vi "Special_Processing.vi"(6 "cluster in":T1, 8 "error in (no error)":errorcluster, 9 "Terminal Map In":map{string, T3}(c390), 10 "Wires":T2[](array[typedef]), 11 "GrowableObjectFunction in":refnum<class "PropertyNode.lvclass">) -> (0 "error out":errorcluster, 1 "Terminal Map Out":map{string, T3}(c390), 2 "Wires out":T2[](array[typedef]), 3 "GrowableObjectFunction out":refnum<class "PropertyNode.lvclass">)   [LabVIEW 2025, in "PropertyNode.lvclass"]
uses:
  PropertyNode.lvclass
  wire.ctl
  Terminal.ctl
  bd.ctl
  Node/Node.lvclass
  Node/Node.lvclass/Node.ctl
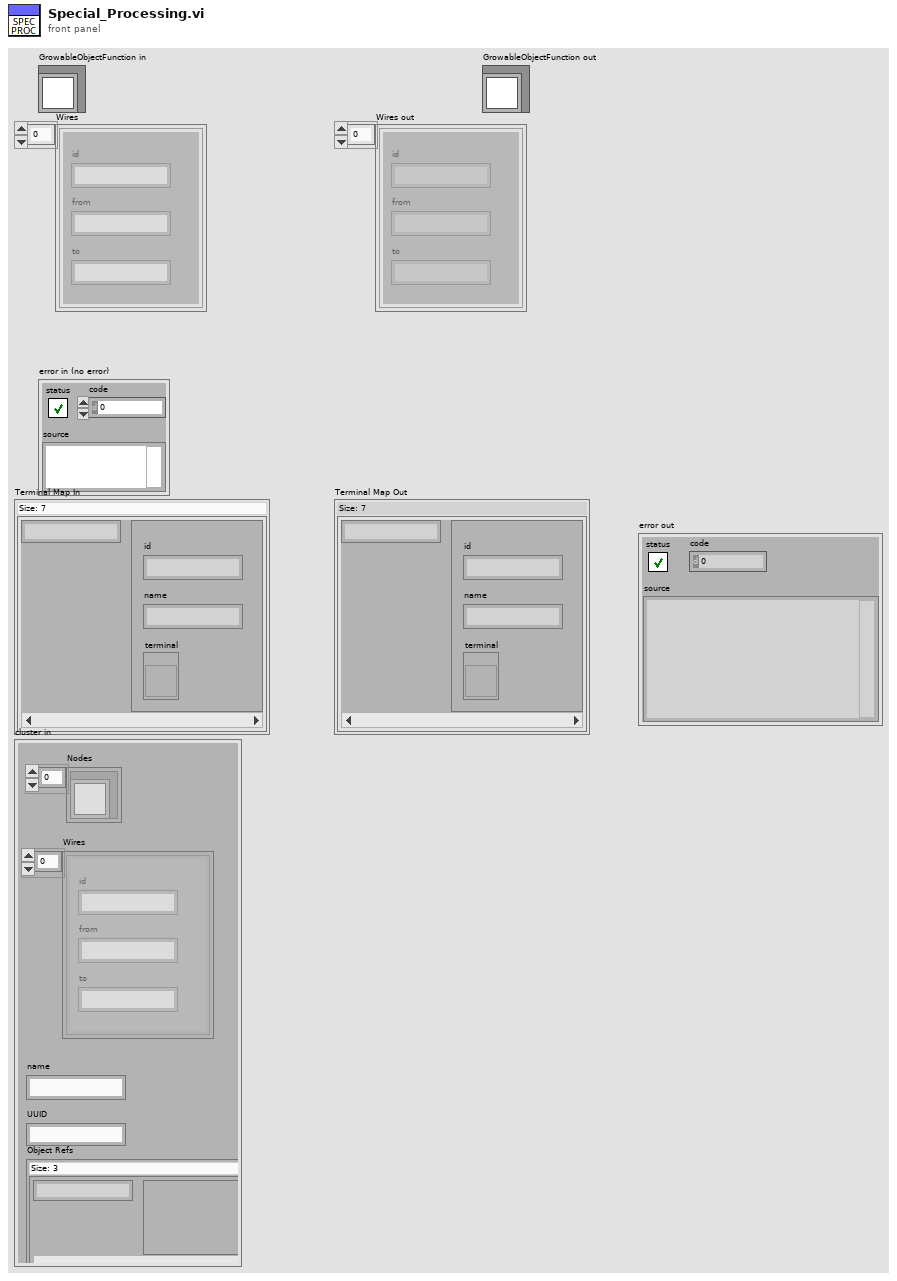
[diagram p1: front panel]
types:
  T1 = typedef "bd.ctl" = cluster{"Nodes":refnum<class "Node.lvclass">[], "Wires":T2[], "name":string, "UUID":string, "Object Refs":map{string, variant}}
  T2 = typedef "wire.ctl" = cluster{"id":string, "from":string, "to":string}
  T3 = typedef "Terminal.ctl" = cluster{"id":string, "name":string, "terminal":refnum<vi>}
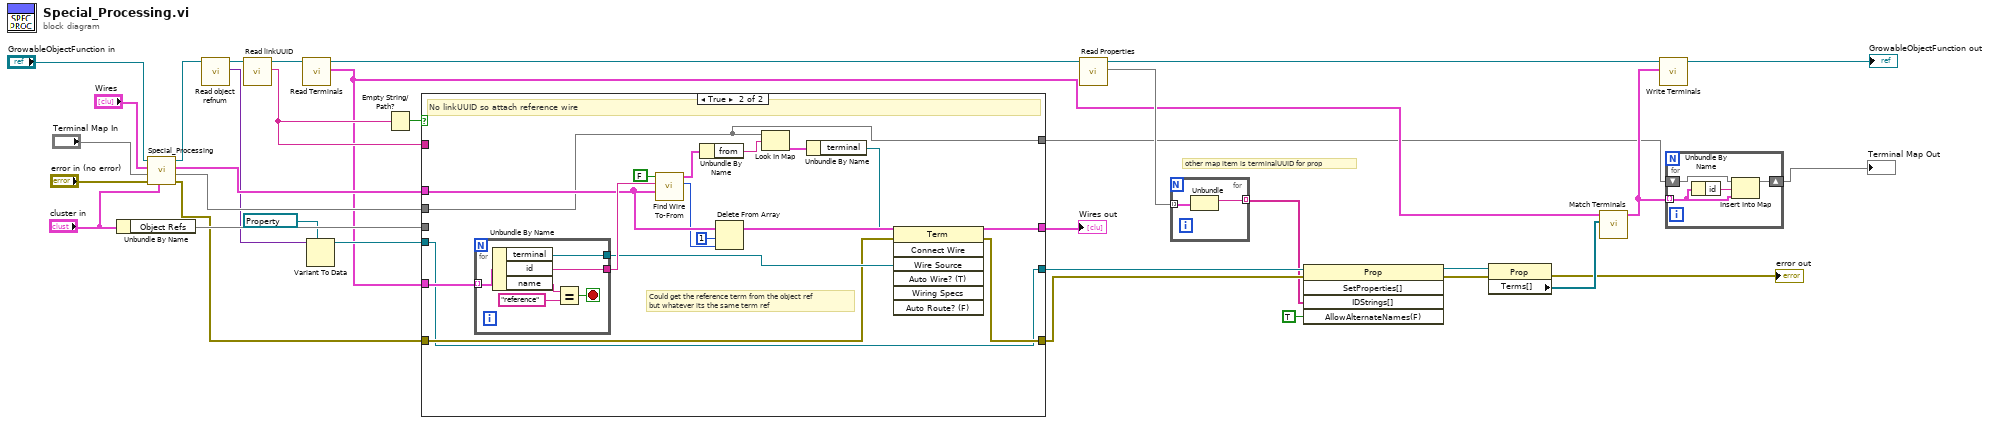
[diagram p0: block diagram]
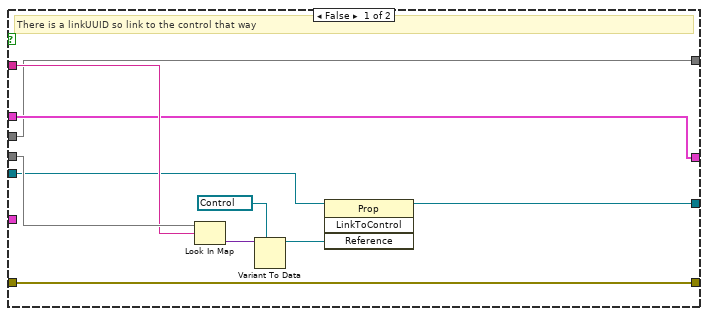
[diagram p2: hidden frame]
diagram:
  # "other map item is terminalUUID for prop"
  n1 = Unbundle By Name("cluster in") -> ("Object Refs"=w26:map{string, variant})
  n2 = call-parent "Special_Processing.vi"("cluster in"="cluster in", "error in (no error)"="error in (no error)", "Terminal Map In"="Terminal Map In", "Wires"="Wires", "Node in"="GrowableObjectFunction in") -> ("error out"=w19:errorcluster, "Terminal Map Out"=w20:map{string, T3}, "Wires out"=w23:T2[], "Node out"=w34:refnum<class "PropertyNode.lvclass">)  [unwired: 3 in]
  n3 = call-dynamic "Read object refnum.vi"("Node in"=w34) -> ("object refnum"=w15:variant, "Node out"=w29:refnum<class "PropertyNode.lvclass">)  [unwired: 8 in, 1 out]
  n4 = call-dynamic "Read linkUUID.vi"("GrowableObjectFunction in"=w29) -> ("linkUUID"=w25:string, "GrowableObjectFunction out"=w28:refnum<class "PropertyNode.lvclass">)  [unwired: 8 in, 1 out]
  n5 = call "Read Terminals.vi"("Node in"=w28) -> ("Terminals"=w8:T3[], "Node out"=w22:refnum<class "PropertyNode.lvclass">)  [unwired: 8 in, 1 out]
  n6 = Variant To Data(type=refnum<vi> refnum ("reference"), Variant=w15) -> (data=w16:refnum<vi>)  [unwired: 1 in, 1 out]
  n7 = Empty String/Path?(string/path=w25) -> (empty?=w27:bool)
  n8 = case shown="True" w27 {
    tunnel: w26 -> [w44 _]
    tunnel: w25 -> [w43 _]
    tunnel: w23 -> [w39 w57]
    tunnel: w8 -> [_ w60]
    tunnel: [w39 w54] -> w21
    tunnel: w20 -> [w37 w46]
    tunnel: w19 -> [w38 w48]
    tunnel: [w38 w47] -> w13
    tunnel: [w37 w46] -> w2
    tunnel: w16 -> [w36 w45]
    tunnel: [w35 w45] -> w14
    frame False {
      # "There is a linkUUID so link to the control that way"
      n9 = Look In Map(map=w44, key=w43) -> (value=w42:variant)  [unwired: 1 in, 1 out]
      n10 = Variant To Data(type=refnum<vi> refnum ("Reference"), Variant=w42) -> (data=w40:refnum<vi>)  [unwired: 1 in, 1 out]
      n11 = invoke class="Prop" method="LinkToControl"(reference=w36, "Reference"=w40) -> (reference out=w35:refnum<vi>)  [unwired: 2 in, 3 out]
    }
    frame True {
      # "Could get the reference term from the object ref \nbut whatever its the same term ref"
      # "No linkUUID so attach reference wire"
      n12 = for {
        tunnel: w60 -> [w66] mode=indexing
        tunnel: [w62] -> w59
        tunnel: [w61] -> w49
        stop <- w63 stop-if-true
        n13 = Unbundle By Name(w66) -> ("terminal"=w61:refnum<vi>, "id"=w62:string, "name"=w65:string)
        n14 = Equal?(x=w65, y="reference") -> (x = y?=w63:bool)
      }
      n15 = call "Find Wire To-From.vi"("Wires"=w57, "termUUID"=w59, "From UUID?"=FALSE) -> ("Index"=w56:i32, "Wire"=w53:T2)  [unwired: 7 in]
      n16 = Unbundle By Name(w53) -> ("from"=w52:string)
      n17 = Delete From Array(array=w57, length=1, index=w56) -> (array with subset deleted=w54:T2[])  [unwired: 1 out]
      n18 = Look In Map(map=w46, key=w52) -> (value=w51:T3)  [unwired: 1 in, 1 out]
      n19 = Unbundle By Name(w51) -> ("terminal"=w50:refnum<vi>)
      n20 = invoke class="Term" method="Connect Wire"(reference=w50, error in=w48, "Wire Source"=w49) -> (error out=w47:errorcluster)  [unwired: 4 in, 6 out]
    }
  }
  "Wires out" <- w21
  n21 = call-dynamic "Read Properties.vi"("PropertyNode in"=w22) -> ("Properties"=w12:map{string, string}, "PropertyNode out"=w18:refnum<class "PropertyNode.lvclass">)  [unwired: 8 in, 1 out]
  n22 = for {
    tunnel: w12 -> [w68] mode=indexing
    tunnel: [w67] -> w11 mode=indexing
    n23 = Unbundle(w68) -> (w67:string)  [unwired: 1 out]
  }
  n24 = invoke class="Prop" method="SetProperties[]"(reference=w14, error in=w13, "IDStrings[]"=w11, "AllowAlternateNames(F)"=TRUE ("Allow Alternate Names? (F)")) -> (reference out=w9:refnum<vi>, error out=w6:errorcluster)  [unwired: 1 in, 3 out]
  n25 = property class="Prop"(reference=w9, error in=w6) -> (error out=→"error out":errorcluster, "Terms[]"=w7:refnum<vi>[])  [unwired: 1 out]
  n26 = call "Match Terminals.vi"("Terms[]"=w7, "Terminals"=w8) -> ("Terminals Out"=w3:T3[])  [unwired: 9 in]
  n27 = call "Write Terminals.vi"("Terminals"=w3, "Node in"=w18) -> ("Node out"=→"GrowableObjectFunction out":refnum<class "PropertyNode.lvclass">)  [unwired: 8 in, 1 out]
  n28 = for {
    shift-right: [w71] -> w1
    shift-left: w2 -> [w72]
    tunnel: w3 -> [w70] mode=indexing
    n29 = Unbundle By Name(w70) -> ("id"=w69:string)
    n30 = Insert Into Map(map in=w72, key=w69, value=w70) -> (map out=w71:map{string, T3})  [unwired: 2 out]
  }
  "Terminal Map Out" <- w1
